vi "DiagnosticsH1R.vi"(7 "Intergation time":dbl=105.0, 9 "Array 2":dbl[][](array[numeric]), 10 "Update previous array?":bool, 11 "Array 1":dbl[][](array[numeric])=array1024x1024[1048576 elements]) -> (0 "RMS subtr ADU  (raw)":dbl=50.01795386315109 format="%#.2f", 1 "mean subtracted ADU (raw)":dbl=11.972700119018555 format="%#.2f", 2 "Median (ADU/sec)":dbl=6.0 format="%#_3f", 3 "Histogram Graph":T4(graph)=[{"X Values"=[-198.0, -194.0, -190.0, -186.0, -182.0, -178.0, -174.0, -170.0, -166.0, -162.0, -158.0, -154.0, -150.0, -146.0, -142.0, -138.0, -134.0, -130.0, -126.0, -122.0, -118.0, -114.0, -110.0, -106.0, -102.0, -98.0, -94.0, -90.0, -86.0, -82.0, -78.0, -74.0, -70.0, -66.0, -62.0, -58.0, -54.0, -50.0, -46.0, -42.0, -38.0, -34.0, -30.0, -26.0, -22.0, -18.0, -14.0, -10.0, -6.0, -2.0, 2.0, 6.0, 10.0, 14.0, 18.0, 22.0, 26.0, 30.0, 34.0, 38.0, 42.0, 46.0, 50.0, 54.0, 58.0, 62.0, 66.0, 70.0, 74.0, 78.0, 82.0, 86.0, 90.0, 94.0, 98.0, 102.0, 106.0, 110.0, 114.0, 118.0, 122.0, 126.0, 130.0, 134.0, 138.0, 142.0, 146.0, 150.0, 154.0, 158.0, 162.0, 166.0, 170.0, 174.0, 178.0, 182.0, 186.0, 190.0, 194.0, 198.0], "Histogram: h(x)"=[0, 0, 0, 0, 0, 0, 0, 0, 0, 0, 0, 0, 0, 0, 0, 0, 0, 0, 0, 0, 0, 0, 0, 0, 0, 0, 0, 0, 1, 2, 5, 13, 30, 65, 138, 280, 543, 1012, 1810, 3105, 5111, 8070, 12228, 17775, 24791, 33174, 42592, 52467, 62009, 70316, 76501, 79856, 79977, 76850, 70851, 62671, 53188, 43309, 33835, 25362, 18239, 12585, 8332, 5292, 3225, 1886, 1058, 569, 294, 146, 69, 32, 14, 6, 2, 1, 0, 0, 0, 0, 0, 0, 0, 0, 0, 0, 0, 0, 0, 0, 0, 0, 0, 0, 0, 0, 0, 0, 0, 0]}, {"X Values"=[-198.0, -194.0, -190.0, -186.0, -182.0, -178.0, -174.0, -170.0, -166.0, -162.0, -158.0, -154.0, -150.0, -146.0, -142.0, -138.0, -134.0, -130.0, -126.0, -122.0, -118.0, -114.0, -110.0, -106.0, -102.0, -98.0, -94.0, -90.0, -86.0, -82.0, -78.0, -74.0, -70.0, -66.0, -62.0, -58.0, -54.0, -50.0, -46.0, -42.0, -38.0, -34.0, -30.0, -26.0, -22.0, -18.0, -14.0, -10.0, -6.0, -2.0, 2.0, 6.0, 10.0, 14.0, 18.0, 22.0, 26.0, 30.0, 34.0, 38.0, 42.0, 46.0, 50.0, 54.0, 58.0, 62.0, 66.0, 70.0, 74.0, 78.0, 82.0, 86.0, 90.0, 94.0, 98.0, 102.0, 106.0, 110.0, 114.0, 118.0, 122.0, 126.0, 130.0, 134.0, 138.0, 142.0, 146.0, 150.0, 154.0, 158.0, 162.0, 166.0, 170.0, 174.0, 178.0, 182.0, 186.0, 190.0, 194.0, 198.0], "Histogram: h(x)"=[196, 191, 188, 180, 195, 222, 218, 216, 218, 231, 236, 240, 225, 261, 258, 269, 280, 258, 282, 336, 343, 334, 390, 401, 416, 549, 549, 609, 687, 867, 867, 1006, 1167, 1377, 1726, 2150, 2736, 3616, 4707, 6132, 8430, 11224, 15066, 20215, 26506, 33802, 42359, 51940, 61443, 70223, 76900, 80333, 80153, 76494, 70797, 62218, 53222, 43312, 33731, 25474, 18058, 12800, 8642, 5579, 3693, 2401, 1531, 1011, 758, 635, 464, 373, 328, 293, 227, 176, 185, 126, 109, 112, 82, 82, 73, 55, 47, 44, 45, 33, 39, 32, 25, 39, 27, 21, 21, 12, 15, 18, 14, 20]}])   [LabVIEW 2012]
uses:
  <vilib>/Analysis/6fits.llb/Curve Fitting Criteria.ctl
  <vilib>/Analysis/baseanly.llb/Mean (DBL).vi
  <vilib>/Analysis/NI_AALPro.lvlib
  <vilib>/gmath/NI_Gmath.lvlib
  <vilib>/Analysis/NI_AALBase.lvlib
panel:
  out "Array size":u16[](array[numeric])
  out "Center":dbl
  out "STDev":dbl
  out "Amplitude":dbl
  out "index of element":i32
  out "Histogram Graph 3":cluster{"X Values":dbl[], dbl[]}(graph)
  in  "method":T1=1 items=["Least Square", "Least Absolute Residual", "Bisquare"]
  out "Hist subtracted":cluster{"X Values":dbl[], dbl[]}(graph)={"X Values"=[-198.0, -194.0, -190.0, -186.0, -182.0, -178.0, -174.0, -170.0, -166.0, -162.0, -158.0, -154.0, -150.0, -146.0, -142.0, -138.0, -134.0, -130.0, -126.0, -122.0, -118.0, -114.0, -110.0, -106.0, -102.0, -98.0, -94.0, -90.0, -86.0, -82.0, -78.0, -74.0, -70.0, -66.0, -62.0, -58.0, -54.0, -50.0, -46.0, -42.0, -38.0, -34.0, -30.0, -26.0, -22.0, -18.0, -14.0, -10.0, -6.0, -2.0, 2.0, 6.0, 10.0, 14.0, 18.0, 22.0, 26.0, 30.0, 34.0, 38.0, 42.0, 46.0, 50.0, 54.0, 58.0, 62.0, 66.0, 70.0, 74.0, 78.0, 82.0, 86.0, 90.0, 94.0, 98.0, 102.0, 106.0, 110.0, 114.0, 118.0, 122.0, 126.0, 130.0, 134.0, 138.0, 142.0, 146.0, 150.0, 154.0, 158.0, 162.0, 166.0, 170.0, 174.0, 178.0, 182.0, 186.0, 190.0, 194.0, 198.0], [196.0, 191.0, 188.0, 180.0, 195.0, 222.0, 217.99999999999997, 215.9999999999999, 217.99999999999926, 230.99999999999562, 235.99999999997513, 239.999999999864, 224.99999999928656, 260.99999999640926, 257.999999982661, 268.99999991966797, 279.99999964291277, 257.99999847706437, 281.9999937682469, 335.99997553414465, 342.9999078422109, 333.9996669379378, 389.99884511228265, 400.9961578365655, 415.9877359649544, 548.9624411395185, 548.889639690847, 608.6888750172159, 686.1584530718424, 864.816047095769, 861.5621193082477, 993.0091503295389, 1137.2239616066067, 1311.5186309768267, 1587.837538557712, 1870.3055496326729, 2192.7507780038404, 2603.6379582093964, 2896.9354227874087, 3026.913078850555, 3319.3642239846777, 3153.5532561654027, 2838.386649751217, 2440.0947180988223, 1714.9815153339368, 627.6120223867547, -233.48175569286104, -526.7845289147735, -566.3855653005667, -92.63182449663873, 398.8761598812853, 477.42830255103763, 176.1845012845297, -356.10550341923954, -54.052301732081105, -453.43198454334924, 33.90846861746104, 2.7489843097282574, -104.17407275528967, 112.34249062430536, -181.3067745689914, 214.7890690785007, 310.289984771478, 286.8850448727608, 467.88007001189726, 515.2507441304506, 473.102727869913, 441.5907396788932, 463.9460411813382, 489.3028650343374, 394.73777016700626, 341.40899786949575, 314.1754242411489, 287.19554165297336, 224.66173859368635, 175.0962550149495, 184.66486466856628, 125.88076163650628, 108.95929635756741, 111.98666871483181, 81.99581078896648, 81.99873696921766, 72.99963464327301, 54.99989859911227, 46.999972998500525, 43.99999310148704, 44.99999830899628, 32.999999602300434, 38.999999910259774, 31.999999980571438, 24.99999999596433, 38.99999999919571, 26.99999999984621, 20.999999999971784, 20.999999999995033, 11.999999999999162, 14.999999999999863, 17.99999999999998, 13.999999999999996, 20.0]}
  out "MEAN  (ADU/sec) AR1":dbl=3.67417049407959 format="%#_3f"
  out "RMS  (ADU/sec) AR1":dbl=182.34897265436433 format="%#_3f"
  out "MEDIAN  subtr ADU  (raw)":dbl=3.0 format="%#.2f"
  out "MEAN  (ADU/sec) Array 2":dbl=-8.298529624938965 format="%#_3f"
  out "RMS (ADU/sec) Array 2":dbl=194.62994975053854 format="%#_3f"
  in  "percent (trim)":dbl=25.0
  out "mean Arr1 ( 2nd method)":dbl=3.67417049407959 format="%0.2f"
  out "mean":dbl=3.67417049407959 format="%0.2f"
  in  "type":T2(ring)
  out "# outside 2":cluster{"total":i32, "below":i32, "above":i32}={"total"=29992, "below"=29383, "above"=609}
  out "Median (ADU/sec) Array 2":dbl=4.0 format="%#_3f"
  out "Histogram Graph 2":T3(graph)={"X Values"=[-198.0, -194.0, -190.0, -186.0, -182.0, -178.0, -174.0, -170.0, -166.0, -162.0, -158.0, -154.0, -150.0, -146.0, -142.0, -138.0, -134.0, -130.0, -126.0, -122.0, -118.0, -114.0, -110.0, -106.0, -102.0, -98.0, -94.0, -90.0, -86.0, -82.0, -78.0, -74.0, -70.0, -66.0, -62.0, -58.0, -54.0, -50.0, -46.0, -42.0, -38.0, -34.0, -30.0, -26.0, -22.0, -18.0, -14.0, -10.0, -6.0, -2.0, 2.0, 6.0, 10.0, 14.0, 18.0, 22.0, 26.0, 30.0, 34.0, 38.0, 42.0, 46.0, 50.0, 54.0, 58.0, 62.0, 66.0, 70.0, 74.0, 78.0, 82.0, 86.0, 90.0, 94.0, 98.0, 102.0, 106.0, 110.0, 114.0, 118.0, 122.0, 126.0, 130.0, 134.0, 138.0, 142.0, 146.0, 150.0, 154.0, 158.0, 162.0, 166.0, 170.0, 174.0, 178.0, 182.0, 186.0, 190.0, 194.0, 198.0], "Histogram: h(x)"=[253, 243, 280, 264, 260, 284, 300, 281, 297, 304, 304, 321, 334, 347, 341, 434, 414, 446, 440, 505, 488, 494, 508, 644, 619, 708, 719, 825, 968, 1009, 1244, 1365, 1638, 1961, 2391, 2832, 3570, 4587, 5840, 7391, 9940, 13190, 17215, 22267, 28530, 35588, 44120, 53662, 62356, 70634, 76007, 78082, 76761, 71806, 65740, 57200, 48371, 38645, 29886, 22190, 15854, 10947, 7238, 4702, 3110, 2098, 1359, 855, 644, 495, 370, 275, 272, 218, 177, 161, 148, 113, 97, 92, 93, 68, 74, 64, 45, 49, 41, 37, 28, 20, 24, 32, 22, 16, 21, 20, 25, 8, 14, 15]}
  out "Median e- (raw)":dbl=18.0 format="%.2f"
  in  "e-/ADU":dbl=1.25
  out "Array previous":dbl[][](array[numeric])
  out "# outside":cluster{"total":i32, "below":i32, "above":i32}={"total"=11160, "below"=10558, "above"=602}
  in  "# bins":i32=100
  in  "min":dbl=-200.0 format="%0.2f"
  in  "max":dbl=200.0 format="%0.2f"
  # "AR1"
  # "Array 2"
  # "Array 1"
  # "A1 - A2"
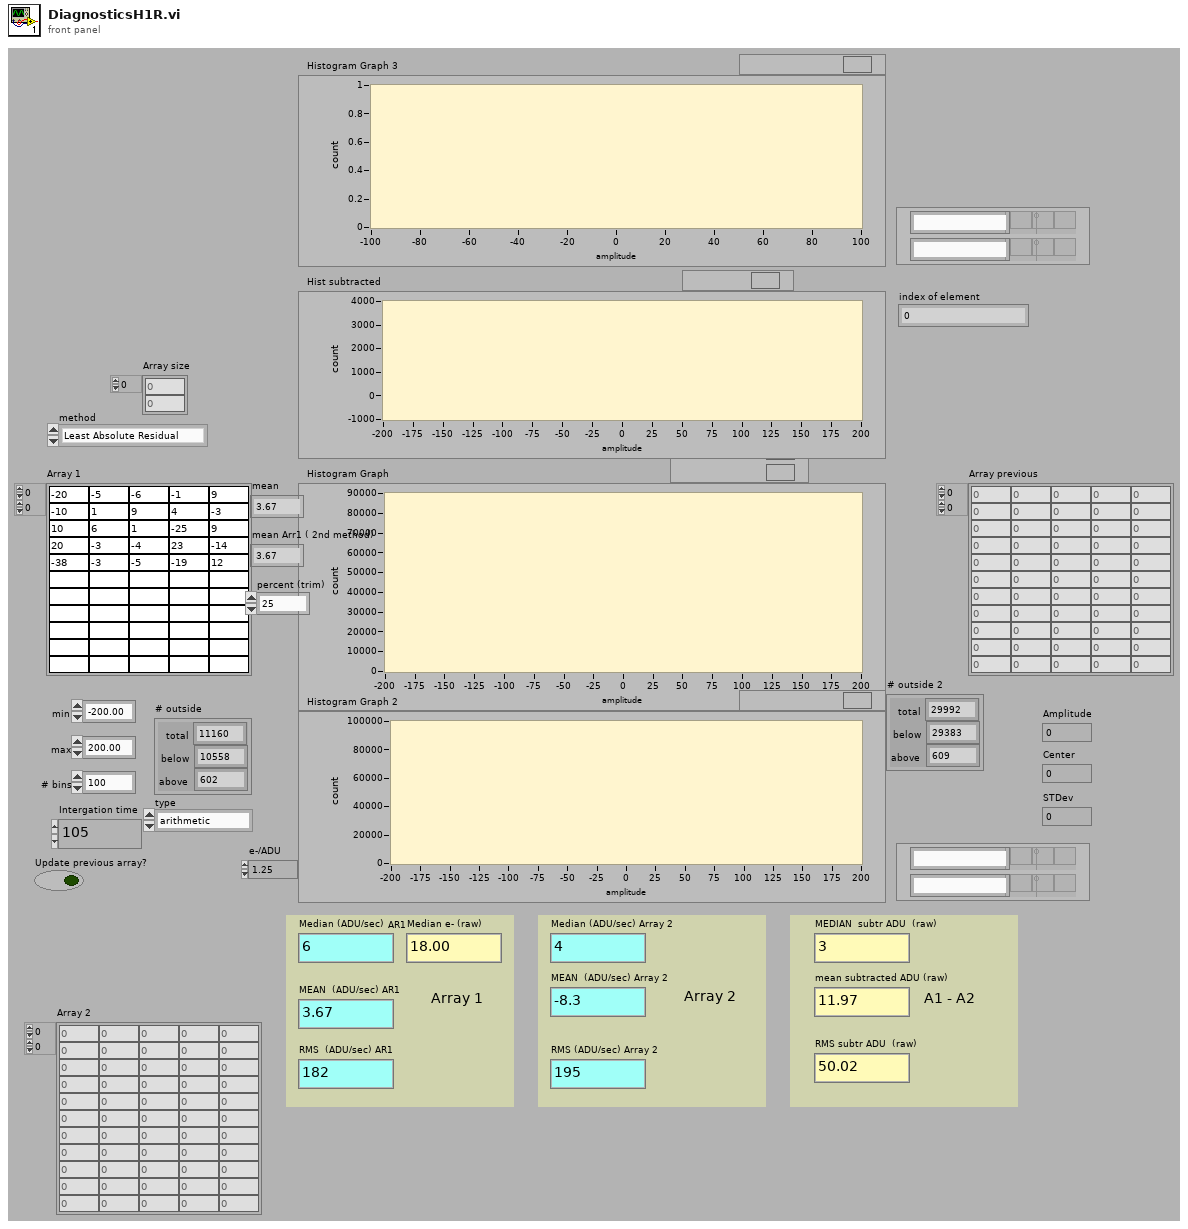
[diagram p1: front panel]
types:
  T1 = typedef "NI_AALPro.lvlib/Curve Fitting Criteria.ctl" = u16
  T2 = enum16{"arithmetic", "geometric", "harmonic", "trimmed", "median"}
  T3 = cluster{"X Values":dbl[], "Histogram: h(x)":i32[]}
  T4 = cluster{"X Values":dbl[], "Histogram: h(x)":i32[]}[]
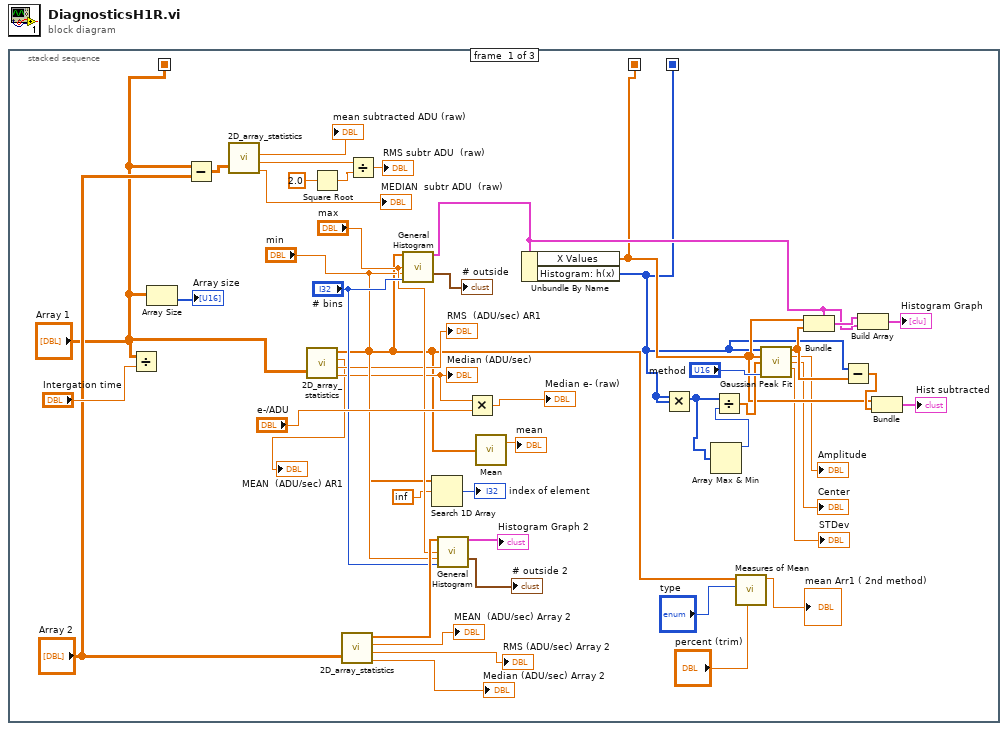
[diagram p0: block diagram]
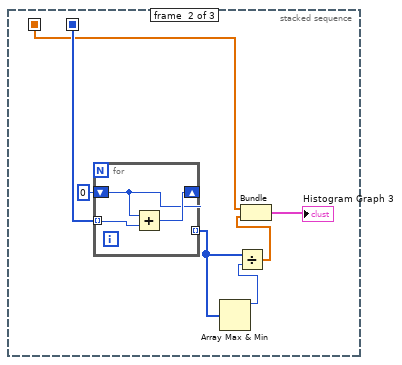
[diagram p2: hidden frame]
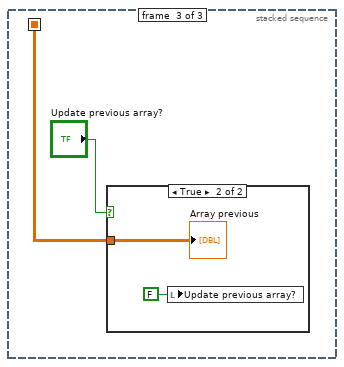
[diagram p3: hidden frame]
diagram:
  n1 = stacked-sequence {
    seq-local: ["Array 1" _ _] -> [_ _ w60]
    seq-local: [w10 _ _] -> [_ w53 _]
    seq-local: [w9 _ _] -> [_ w54 _]
    frame #0 {
      n2 = Divide(x="Array 1", y="Intergation time") -> ()  [unwired: 1 out]
      n3 = Array Size(array="Array 1") -> (size(s)=→"Array size":i32[])
      n4 = Subtract(x="Array 1", y="Array 2") -> (x-y=w28:dbl[][])
      n5 = call "2D_array_statistics.vi"("Array"=w28) -> ("mean 2"=→"mean subtracted ADU (raw)":dbl, "RMS 2"=w32:dbl, "median 3"=→"MEDIAN  subtr ADU  (raw)":dbl)  [unwired: 2 in, 1 out]
      n6 = call "2D_array_statistics.vi"("Array"="Array 1") -> ("1D array"=w6:dbl[], "mean 2"=→"MEAN  (ADU/sec) AR1":dbl, "RMS 2"=→"RMS  (ADU/sec) AR1":dbl, "median 3"=w27:dbl)  [unwired: 2 in]
      "Median (ADU/sec)" <- w27
      n7 = Square Root(x=2.0) -> (sqrt(x)=w31:dbl)
      n8 = call "2D_array_statistics.vi"("Array"="Array 2") -> ("1D array"=w45:dbl[], "mean 2"=→"MEAN  (ADU/sec) Array 2":dbl, "RMS 2"=→"RMS (ADU/sec) Array 2":dbl, "median 3"=→"Median (ADU/sec) Array 2":dbl)  [unwired: 2 in]
      n9 = Divide(x=w32, y=w31) -> (x/y=→"RMS subtr ADU  (raw)":dbl)
      n10 = call <vilib>:"General Histogram.vi"("X"=w6, "max"="max", "min"="min", "# bins"="# bins") -> ("Histogram Graph"=w18:T3, "# outside"=→"# outside":cluster{"total":i32, "below":i32, "above":i32})  [unwired: 7 in, 3 out]
      n11 = Search 1D Array(1D array=w6, element=inf) -> (index of element=→"index of element":i32)  [unwired: 1 in]
      n12 = call <vilib>:"General Histogram.vi"("X"=w45, "max"="max", "min"="min", "# bins"="# bins") -> ("Histogram Graph"=→"Histogram Graph 2":T3, "# outside"=→"# outside 2":cluster{"total":i32, "below":i32, "above":i32})  [unwired: 7 in, 3 out]
      n13 = Multiply(x=w27, y="e-/ADU") -> (x*y=→"Median e- (raw)":dbl)
      n14 = call-poly <vilib>:"Mean.vi"("X"=w6) -> ("mean"=→"mean":dbl)  [unwired: 1 out]
      n15 = Unbundle By Name(w18) -> ("X Values"=w10:dbl[], "Histogram: h(x)"=w9:i32[])
      n16 = Multiply(x=w9, y=w9) -> (x*y=w12:i32[])
      n17 = Array Max & Min(array=w12) -> (max value=w11:i32)  [unwired: 3 out]
      n18 = Divide(x=w12, y=w11) -> (x/y=w13:dbl[])
      n19 = call <vilib>:"Measures of Mean.vi"("percent (trim)"="percent (trim)", "type"="type", "x array"=w6) -> ("mean value"=→"mean Arr1 ( 2nd method)":dbl)  [unwired: 7 in, 1 out]
      n20 = call <vilib>:"Gaussian Peak Fit.vi"("Y"=w9, "X"=w10, "Weight"=w13, "method"="method") -> ("Best Gaussian Fit"=w17:dbl[], "amplitude"=→"Amplitude":dbl, "center"=→"Center":dbl, "standard deviation"=→"STDev":dbl)  [unwired: 5 in, 3 out]
      n21 = Bundle(cluster=w18, "X Values"=w10, "Histogram: h(x)"=w17) -> (w19:T3)
      n22 = Subtract(x=w9, y=w17) -> (x-y=w16:dbl[])
      n23 = Build Array(w19, w18) -> (→"Histogram Graph":T4)
      n24 = Bundle("X Values"=w10, w16) -> (→"Hist subtracted":cluster{"X Values":dbl[], dbl[]})  [unwired: 1 in]
    }
    frame #1 {
      n25 = for {
        tunnel: w54 -> [w58] mode=indexing
        shift-right: [w57] -> _
        shift-left: 0 -> [w56]
        tunnel: [w56] -> w51 mode=indexing
        n26 = Add(x=w56, y=w58) -> (x+y=w57:i32)
      }
      n27 = Array Max & Min(array=w51) -> (max value=w50:i32)  [unwired: 3 out]
      n28 = Divide(x=w51, y=w50) -> (x/y=w49:dbl[])
      n29 = Bundle("X Values"=w53, w49) -> (→"Histogram Graph 3":cluster{"X Values":dbl[], dbl[]})  [unwired: 1 in]
    }
    frame #2 {
      n30 = case shown="True" "Update previous array?" {
        tunnel: w60 -> [_ w62]
        frame False {
        }
        frame True {
          n31 = local write "Update previous array?"(FALSE ("Update previous array?")) -> ()
          "Array previous" <- w62
        }
      }
    }
  }
